vi "test - read Cluster From Session.vi"(8 "error in (no error)":errorcluster, 11 "TestCase in":refnum<class "csm-ini-variable-addon.lvclass">) -> (0 "error out":errorcluster, 3 "TestCase out":refnum<class "csm-ini-variable-addon.lvclass">)   [LabVIEW 2017, in "csm-ini-variable-addon.lvclass"]
uses:
  csm-ini-variable-addon.lvclass
  70d35eaa-da7f-49f1-8782-b29d93c4b83f.vi
  70d35eaa-da7f-49f1-8782-b29d93c4b83f.vi/99de0c97-112a-4c86-9094-c187659127e1.vi
  <userlib>/_NEVSTOP/Communicable State Machine(CSM)/Utility/Build Error Cluster.vi
  <vilib>/Utility/Data Type/Get Type Information.vi
  <userlib>/_NEVSTOP/Communicable State Machine(CSM)/addons/API-String-Arugments-Support/_Support/Data To SingleElementsArray_csm.vi
  <userlib>/_NEVSTOP/Communicable State Machine(CSM)/addons/API-String-Arugments-Support/_Support/Data To API String Arguments.vi
  INI-Static-Variable-Support/_Support/Parse Used Session and Name.vi
  INI-Static-Variable-Support/_Support/INI-FGV.vi
  INI-Static-Variable-Support/_Support/Populate String with INI Variable.vi
  <userlib>/_NEVSTOP/Communicable State Machine(CSM)/addons/API-String-Arugments-Support/_Support/Convert API String Arguments to Data(variant).vi
  <userlib>/_NEVSTOP/Communicable State Machine(CSM)/addons/API-String-Arugments-Support/_Support/SingleElementsArray To Data_csm.vi
  <vilib>/addons/_JKI Toolkits/VI Tester/TestCase.llb/TestCase.lvclass
  C:/Program Files (x86)/National Instruments/LabVIEW 2017/vi.lib/addons/_JKI Toolkits/VI Tester/TestCase.llb/TestCase.lvclass
panel:
  out "Array":cluster{"Type":string, "path ":string}[](array[cluster])
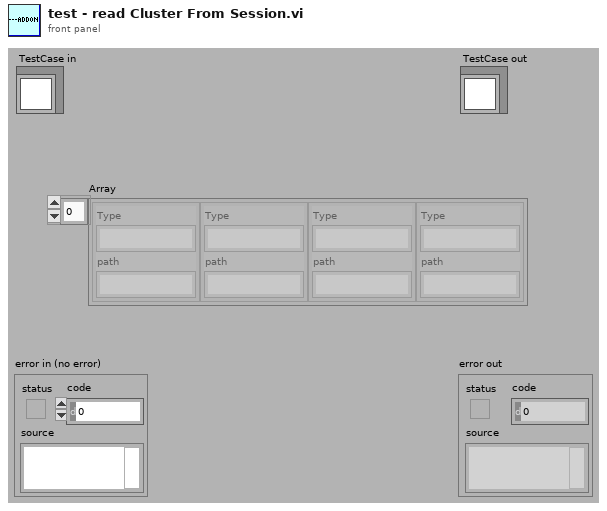
[diagram p1: front panel]
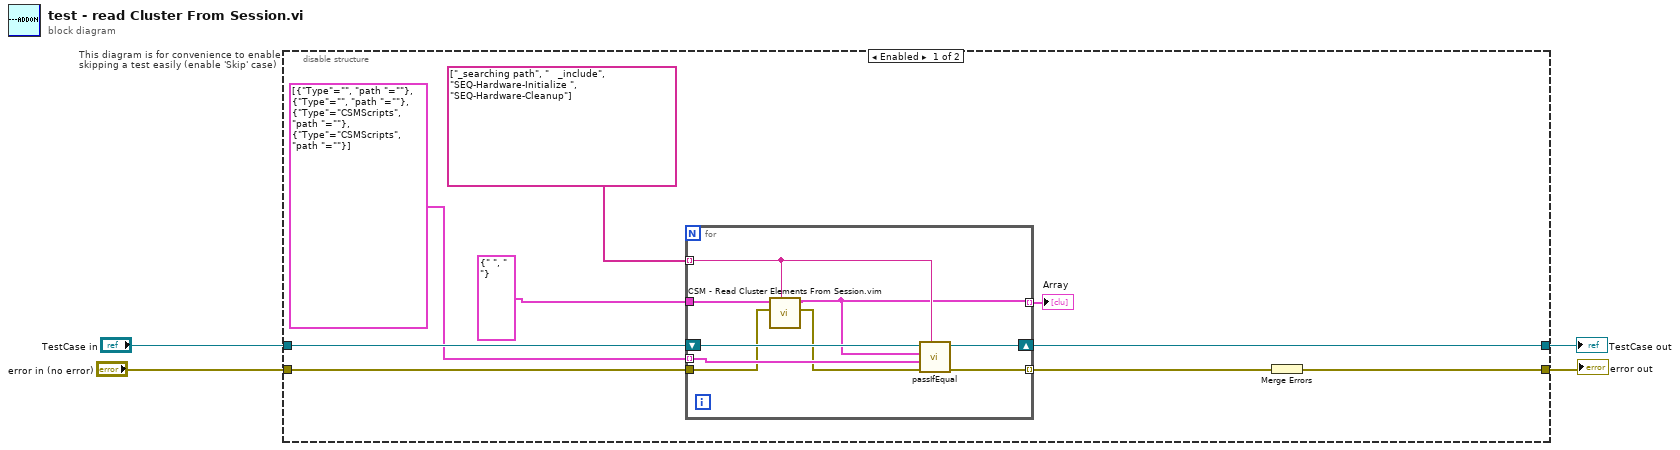
[diagram p0: block diagram]
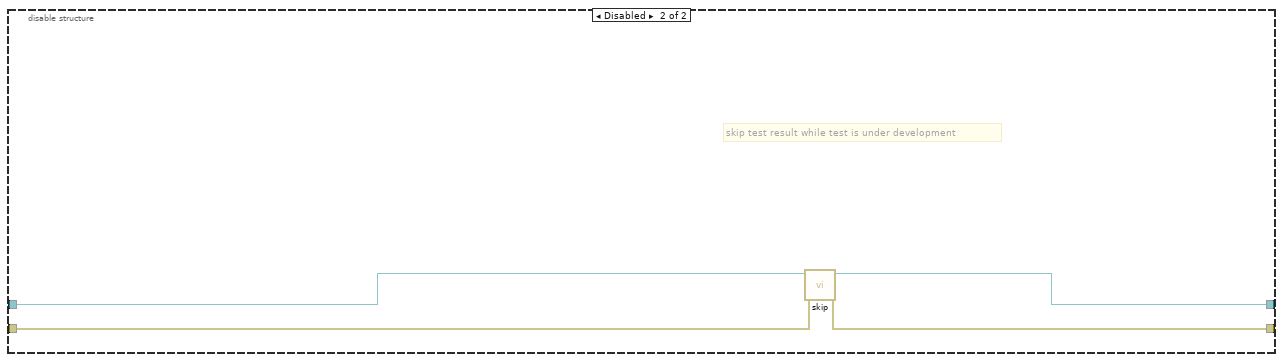
[diagram p2: hidden frame]
diagram:
  n1 = disable-structure "This diagram is for convenience to enable skipping a test easily (enable 'Skip' case)" shown="Enabled" {
    disable-tunnel: "TestCase in" -> [w10 w26]
    disable-tunnel: [w13 w24] -> w1
    disable-tunnel: [w5 w25] -> w3
    disable-tunnel: "error in (no error)" -> [w11 w23]
    frame Enabled {
      n2 = for {
        shift-right: [w22] -> w13
        shift-left: w10 -> [w20]
        tunnel: cluster{"Type":string, "path ":string} {"Type"=" ", "path "=" "} -> [w19]
        tunnel: string[] ["_searching path", "   _include", "SEQ-Hardware-Initialize ", "SEQ-Hardware-Cleanup"] ("Section Name(\"\" as Default)") -> [w17] mode=indexing
        tunnel: cluster{"Type":string, "path ":string}[] [{"Type"="", "path "=""}, {"Type"="", "path "=""}, {"Type"="CSMScripts", "path "=""}, {"Type"="CSMScripts", "path "=""}] -> [w18] mode=indexing
        tunnel: [w16] -> w6 mode=indexing
        tunnel: w11 -> [w15]
        tunnel: [w21] -> w12 mode=indexing
        n3 = call "CSM - Read Cluster Elements From Session.vim"("Section Name(\"\" as Default)"=w17, "error in (no error)"=w15, "Cluster"=w19) -> ("error out"=w14:errorcluster, "Cluster out"=w16:cluster{"Type":string, "path ":string})  [unwired: 5 in]
        n4 = call-dynamic "passIfEqual.vi"("custom report message (\"\")"=w17, "error in (no error)"=w14, "y"=w18, "x"=w16, "TestCase in"=w20) -> ("error out"=w21:errorcluster, "TestCase out"=w22:refnum<class "csm-ini-variable-addon.lvclass">)  [unwired: 5 in]
      }
      "Array" <- w6
      n5 = Merge Errors(w12) -> (w5:errorcluster)
    }
    frame Disabled {
      # "skip test result while test is under development"
      n6 = call <vilib>:"skip.vi"("error in (no error)"=w23, "TestCase in"=w26) -> ("error out"=w25:errorcluster, "TestCase out"=w24:refnum<class "csm-ini-variable-addon.lvclass">)  [unwired: 8 in]
    }
  }
  "error out" <- w3
  "TestCase out" <- w1
